vi "Trajectory Box Monitor.vi"() -> ()   [LabVIEW 2017]
uses:
  TCP/TCP Host/Controls/Host- Queue States.ctl
  TCP/TCP Host/Controls/Control - Testscreen.ctl
  Controls/Testscreen_Input cluster.ctl
  <vilib>/addons/database/Connection.llb/Conn ObjectReference.ctl
  Controls/Network_states.ctl
  TCP/TCP Engine/Controls/TCP - Driver Control.ctl
  Variable/Global 1.vi
  <vilib>/addons/database/Connection.llb/DB Tools Open Connec (String).vi
  <vilib>/addons/database/NI_Database_API.lvlib
panel:
  out "error out":errorcluster
  out "array":string[](array[string])
  out "Test Running":bool
  in  "DataLog Duration":string="00:01:27"
  in  "Exit":bool
  in  "Report":bool
  in  "Settings":bool
  in  "Test Screen":bool
  in  "ID Status":string
  in  "?":enum32{"Option A", "Option B"}(tab)
  in  "Test Profile":T1(array[cluster])=[{"Ram Up Time"=10.0, "Hold Time"=5.0, "Ramp Down"=10.0, "Concentration Value"=25.0}, {"Ram Up Time"=15.0, "Hold Time"=10.0, "Ramp Down"=5.0, "Concentration Value"=35.0}, {"Ram Up Time"=0.0, "Hold Time"=0.0, "Ramp Down"=0.0, "Concentration Value"=0.0}]
  out "Profile Plotting":cluster{"X":dbl, "Y":dbl}[](graph)
  in  "Profile File Selection":u16(ring) items=["Test A", "Test B", "Test C"]
  in  "Iterations":dbl
  in  "Gas Selection":u16(ring) items=["Test A", "Test B", "Test C"]
  in  "Drive  2":string
  in  "Drive":string
  in  "IP Address":string
  in  "error in (no error)":errorcluster
  in  "Note":string
  in  "Tab- Main":enum32{"Settings", "Report", "Testscreen"}(tab)
  in  "Tab Control Testscreen 4":enum32{"Channel Mapping", "Test Settings"}(tab)
  in  "Channel Mapping":T2(array[cluster])
  in  "Sampling Frequency (Hz)":string="Trajectory"
  in  "Wifi Name":string="Trajectory"
  in  "Test Inactivity Time":dbl=30.0 format="%<%H:%M:%S>t"
  in  "Drive Path":path=path "D:/Trajectory Data"
  in  "cRIO IP Address":string="192.168.1.1"
  out "Test Time":dbl=1.0 format="%<%H:%M:%S>t"
  in  "Save Test Settings":bool
  in  "Tab Control Testscreen 5":enum32{"Report", "Detailed Report"}(tab)
  in  "Fetch Report":bool
  in  "To Date & Time":timestamp format="%<%x>T"
  in  "From Date & Time":timestamp format="%<%x>T"
  out "Report Data":i32(listbox)
  in  "Test Stop Time :":string="12:59:05"
  in  "Tab Control Testscreen 6":enum32{"Data", "Histogram"}(tab)
  in  "Report Data 2":i32(listbox)
  out "XY Graph 3":cluster{i32, "Numeric":u16}[](graph)
  in  "ID Status :":string="00068OK"
  in  "ID :":string="Trajectory"
  in  "Angle :":string="Multi"
  in  "Flow :":string="Flow"
  in  "Material :":string="Cole"
  in  "Furnace :":string="G Furnace"
  in  "Test Start Time:":string="12:59:05"
  in  "Date :":string="02/07/2021"
  out "Date":string
  in  "Tab- Main 2":T3(tab)
  in  "Test details":T4={"Furnace"="Furnace A", "Material"="Coke", "Angle"="Multi Angle", "ID"="Trajectory 9", "Flowrate"="Flow", "Test Name"="Coke Burn", "Tested By"="Anirban"}
  in  "Save Test Info":bool
  out "Data Logging Path":path
  in  "Probe 2":bool[](array[boolean])=[TRUE, FALSE, FALSE, FALSE, TRUE, FALSE, FALSE, FALSE, FALSE, FALSE, FALSE, FALSE, FALSE, FALSE, FALSE, FALSE, FALSE, FALSE, FALSE, FALSE, FALSE, FALSE, FALSE, FALSE, FALSE, FALSE, FALSE, FALSE, FALSE, FALSE, FALSE, FALSE, FALSE, FALSE, FALSE, FALSE, FALSE, FALSE, FALSE, FALSE, FALSE, FALSE, FALSE, FALSE, FALSE, FALSE, FALSE, FALSE, FALSE, FALSE, FALSE, FALSE, FALSE, FALSE, FALSE, FALSE, FALSE, FALSE, FALSE, FALSE]
  in  "Probe":bool[](array[boolean])
  in  "Probe 3":bool[](array[boolean])=[TRUE, FALSE, FALSE, FALSE, TRUE, FALSE, FALSE, FALSE, FALSE, FALSE, FALSE, FALSE, FALSE, FALSE, FALSE, FALSE, FALSE, FALSE, FALSE, FALSE, FALSE, FALSE, FALSE, FALSE, FALSE, FALSE, FALSE, FALSE, FALSE, FALSE, FALSE, FALSE, FALSE, FALSE, FALSE, FALSE, FALSE, FALSE, FALSE, FALSE, FALSE, FALSE, FALSE, FALSE, FALSE, FALSE, FALSE, FALSE, FALSE, FALSE, FALSE, FALSE, FALSE, FALSE, FALSE, FALSE, FALSE, FALSE, FALSE, FALSE]
  out "XY Graph":cluster{i32, "Numeric":i32}[](graph)
  in  "Setup":bool
  out "Datalog Duration":dbl format="%<%H:%M:%S>t"
  in  "Disk Space Host":string="Trajectory 9"
  in  "Disk Space cRIO":string="Trajectory 9"
  in  "Calibrations":bool
  in  "Alarms":i32(listbox)
  out "Wifi":bool=TRUE
  out "Logging 3":bool=TRUE
  in  "Start Test":bool
  in  "Stop Test":bool
  out "Message":string="Acquiring Data"
  # "Test Setup Setting"
  # "Trajectory Box Monitor System"
  # "Trajectory Box Monitor"
  # "1"
  # "5"
  # "10"
  # "15"
  # "20"
  # "41"
  # "45"
  # "50"
  # "55"
  # "60"
  # "21"
  # "25"
  # "30"
  # "40"
  # "35"
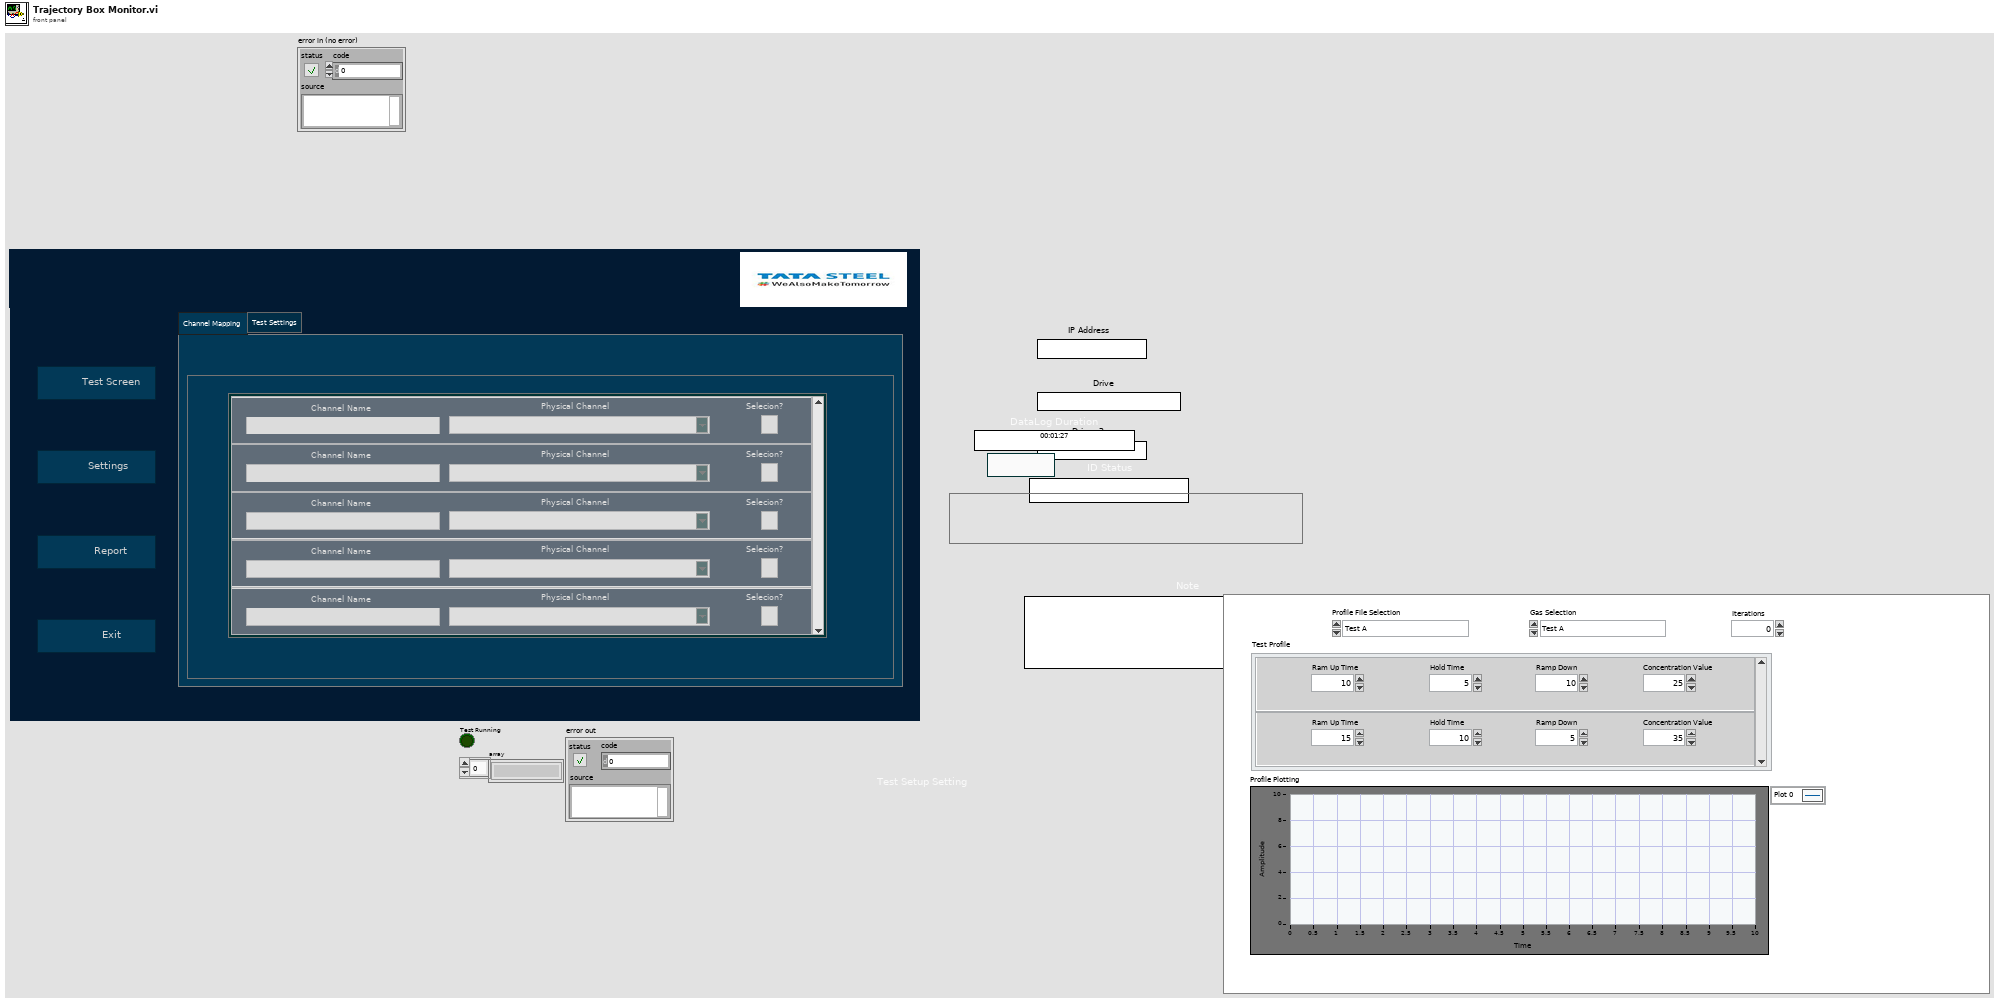
[diagram p1: front panel]
types:
  T1 = cluster{"Ram Up Time":dbl, "Hold Time":dbl, "Ramp Down":dbl, "Concentration Value":dbl}[]
  T2 = cluster{"Channel Name":string, " Physical Channel":tag, "Selecion?":bool}[]
  T3 = enum32{"Test Information", "Sensor Status", "Histogram", "Info", "Software Log"}
  T4 = cluster{"Furnace":string, "Material":string, "Angle":string, "ID":string, "Flowrate":string, "Test Name":string, "Tested By":string}
  T5 = typedef "Network_states.ctl" = enum16{"Connect", "Transfer Files", "Close"}
  T6 = typedef "Testscreen_Input cluster.ctl" = cluster{"Message":string, "Histogram Data":i32[], "Timer 1":u32, "Test Running":bool, "connection reference":T7}
  T7 = typedef "NI_Database_API.lvlib/Conn ObjectReference.ctl" = refnum<k1>
  T8 = typedef "Control - Testscreen.ctl" = enum16{"No Event", "Init", "Download Files", "Test Running", "Update Test Results", "Machine Unhealthy", "Autotest Started", "Test Aborted", "Sequence Complete", "Update Sensor Data", "Log File Available", "Machine Mode", "Aux Logging Started", "Aux File Saved", "Get PID Values", "View Report", "Exit", "Wait", "Abort", "Copy Log File", "Generate Alarm", "Send Test Details"}
  T9 = typedef "Host- Queue States.ctl" = enum16{"Initialize", "Enqueue", "Enqueue Priority", "Dequeue", "Flush", "Destroy"}
  T10 = cluster{"Test details":cluster{"Furnace":string, "Material":string, "Angle":string, "ID":string, "Flowrate":string, "Test Name":string, "Tested By":string}, "Datalog Duration":dbl}
  T11 = typedef "TCP - Driver Control.ctl" = enum16{"Test Settings", "Boolean Commands", "Test Results", "Send Test Details"}
  T12 = cluster{"Channel Name":string, " Physical Channel":tag, "Selecion?":bool}
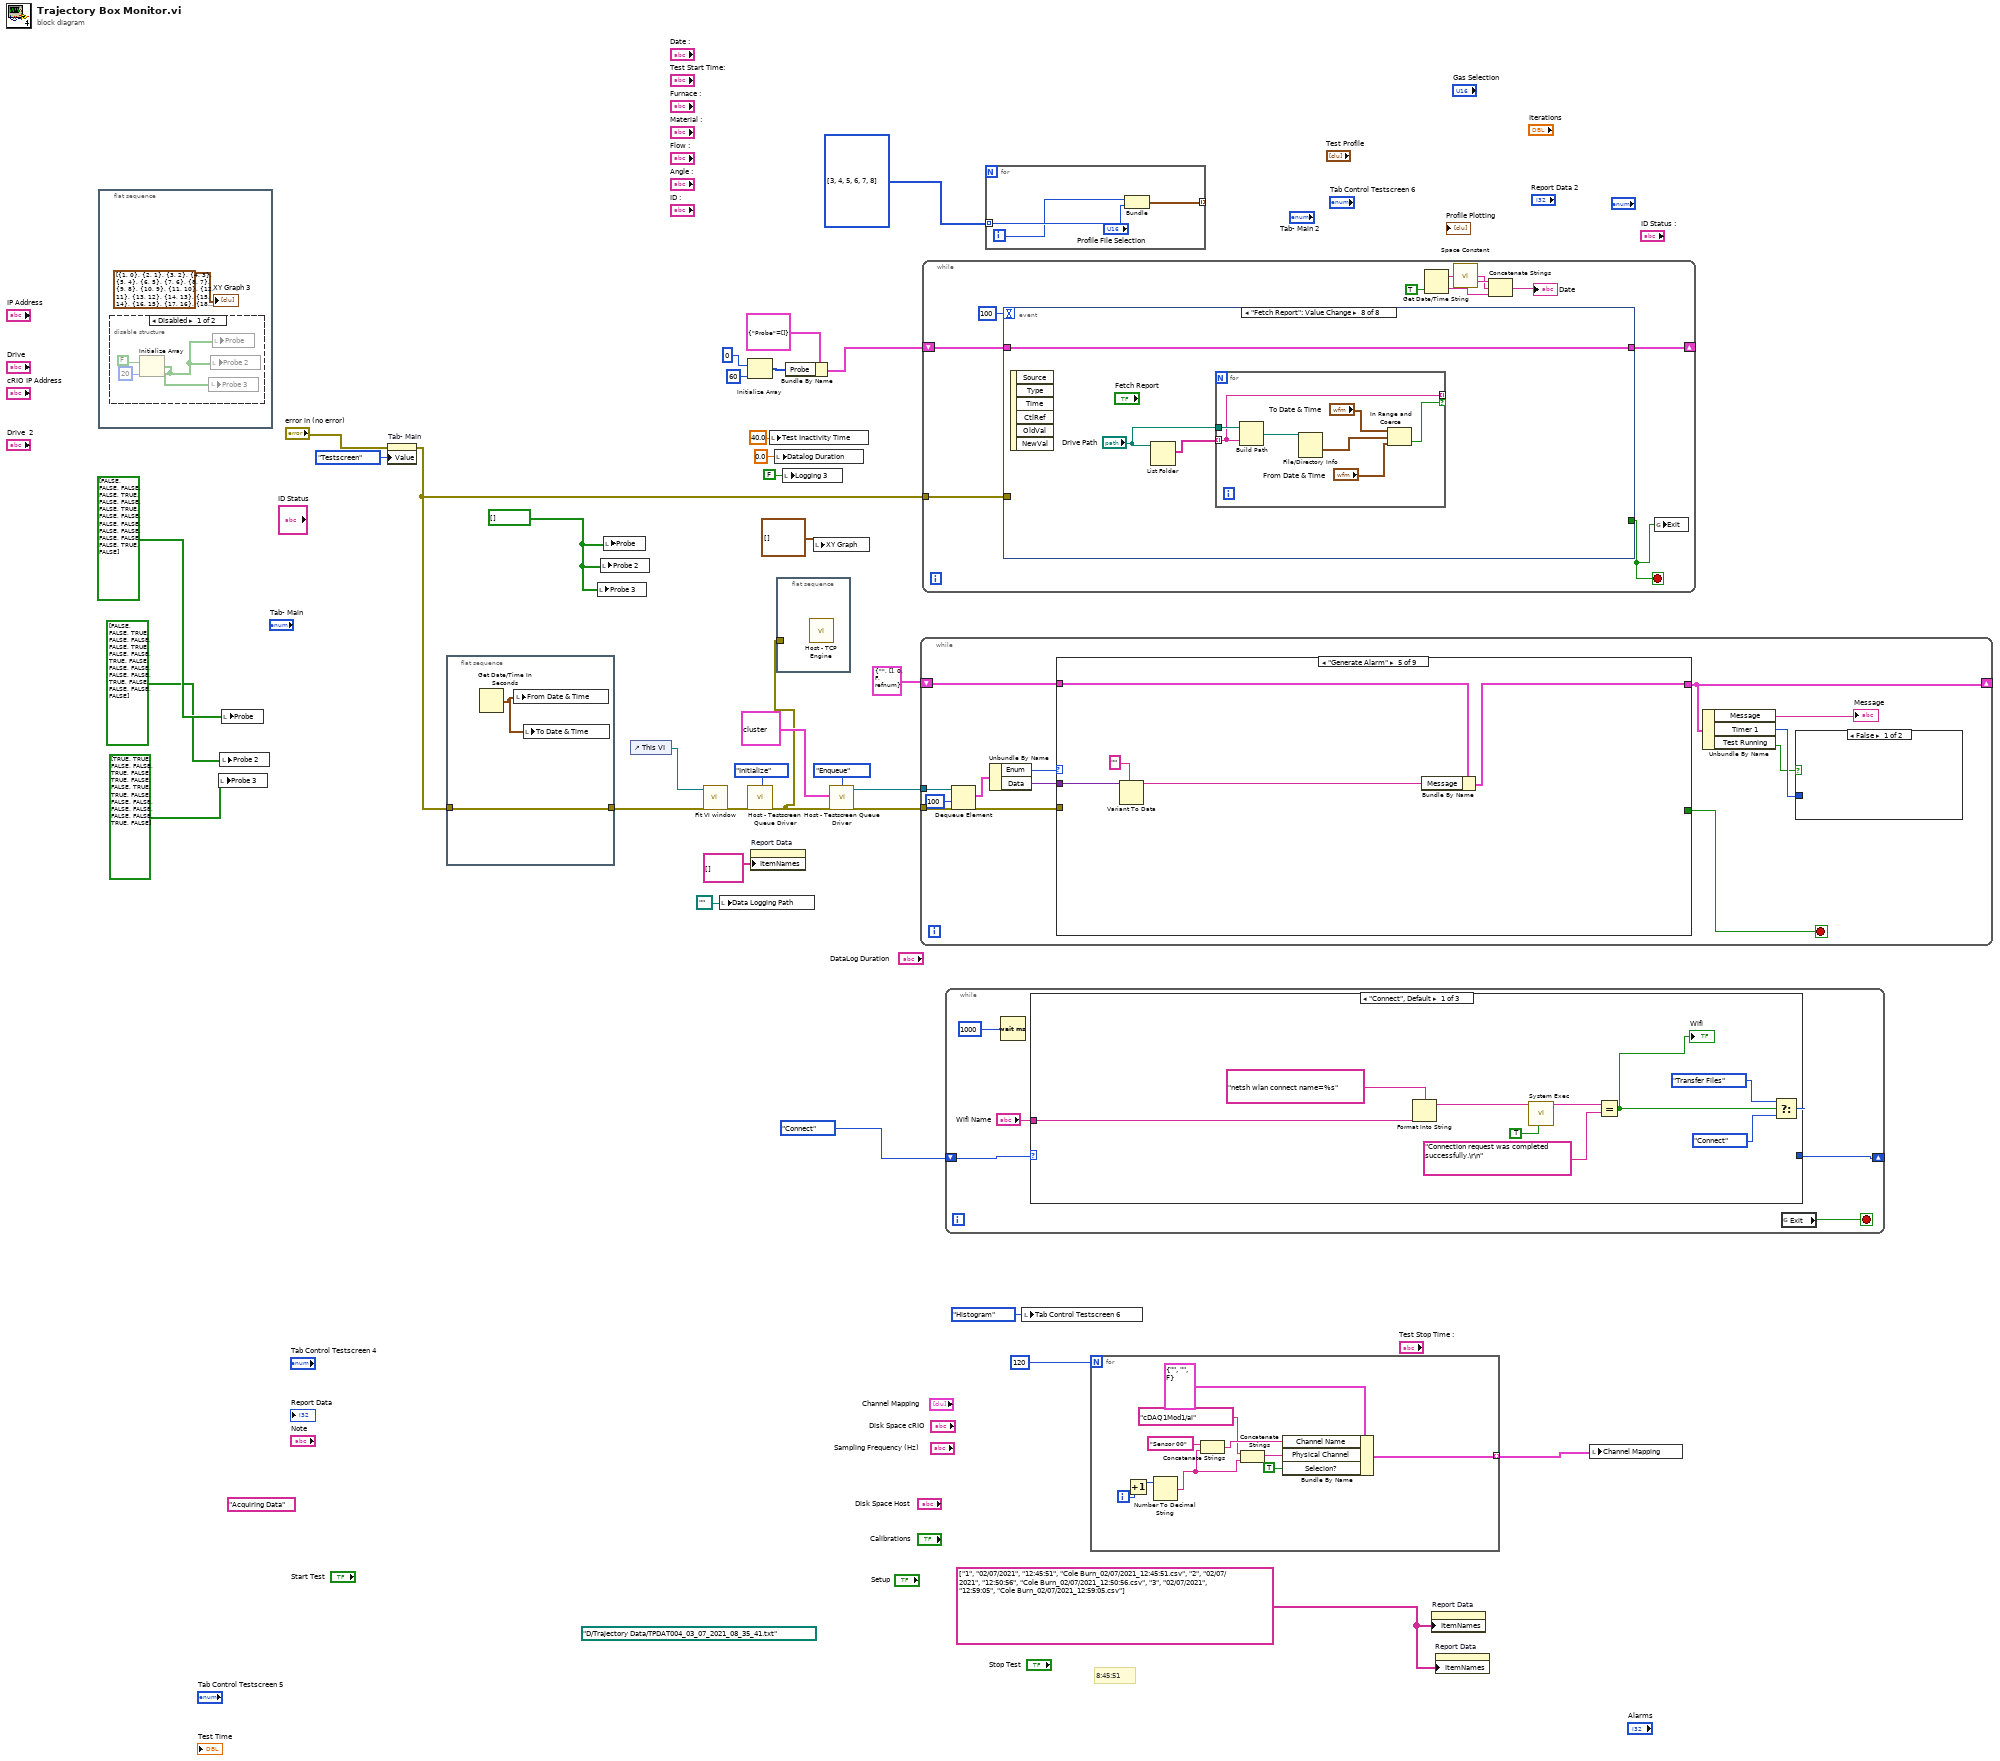
[diagram p0: block diagram]
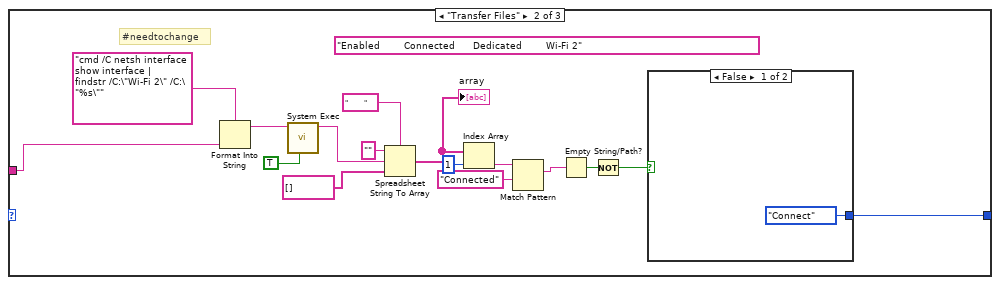
[diagram p2: hidden frame]
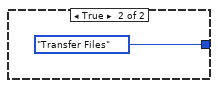
[diagram p3: hidden frame]
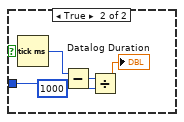
[diagram p5: hidden frame]
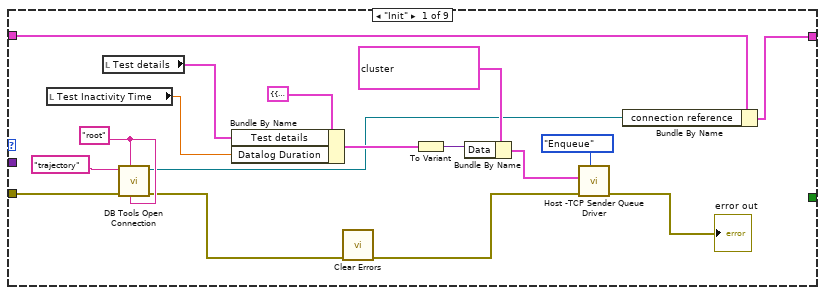
[diagram p6: hidden frame]
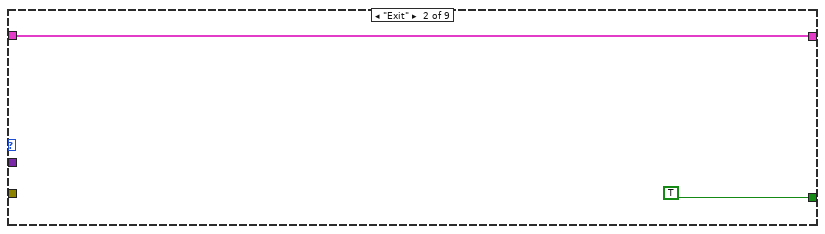
[diagram p7: hidden frame]
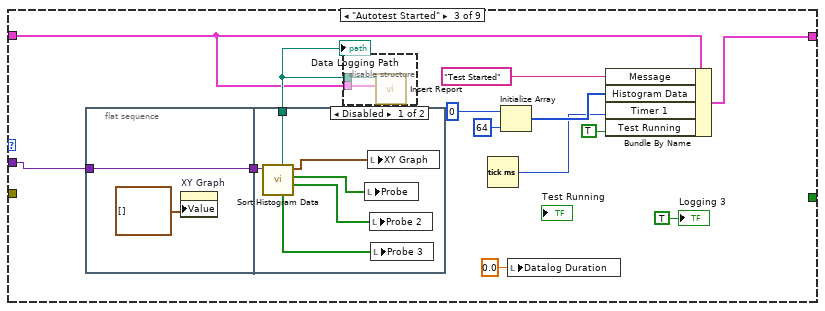
[diagram p8: hidden frame]
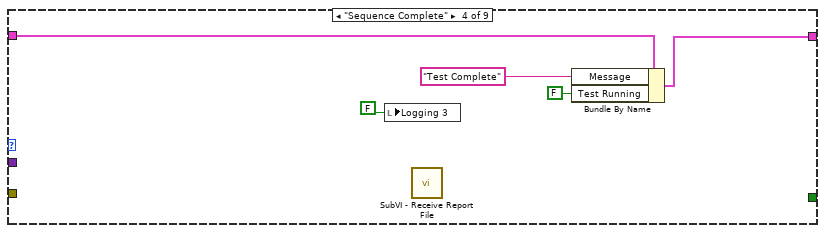
[diagram p10: hidden frame]
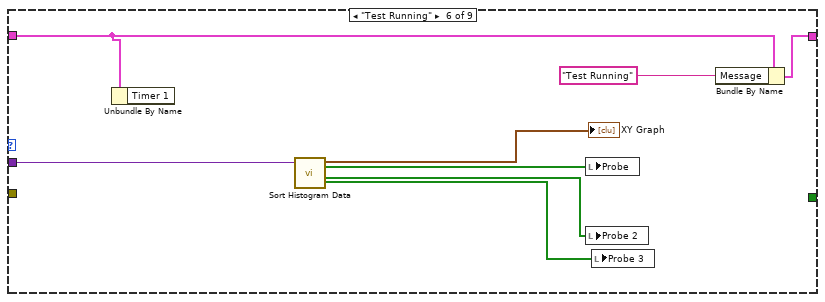
[diagram p11: hidden frame]
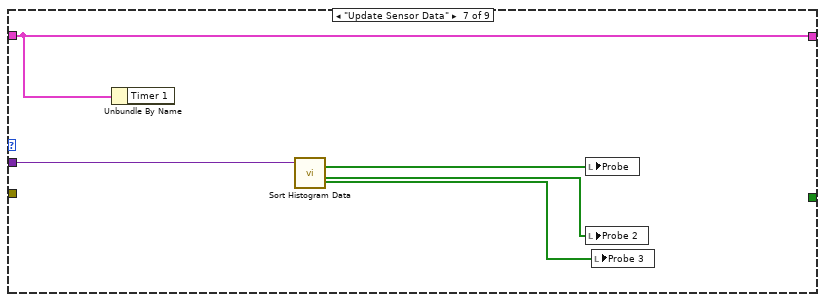
[diagram p12: hidden frame]
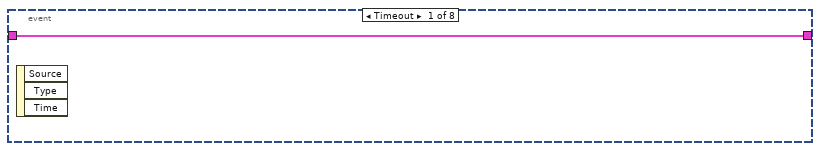
[diagram p16: hidden frame]
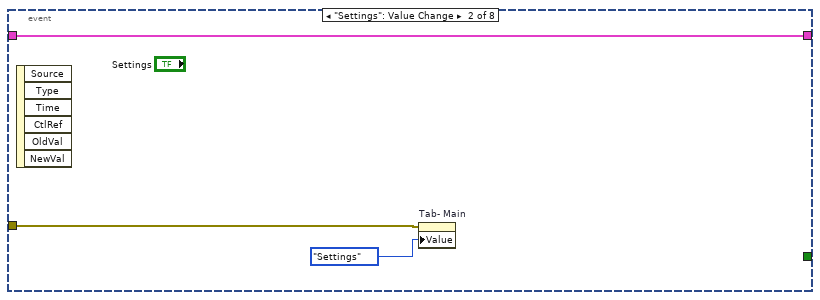
[diagram p17: hidden frame]
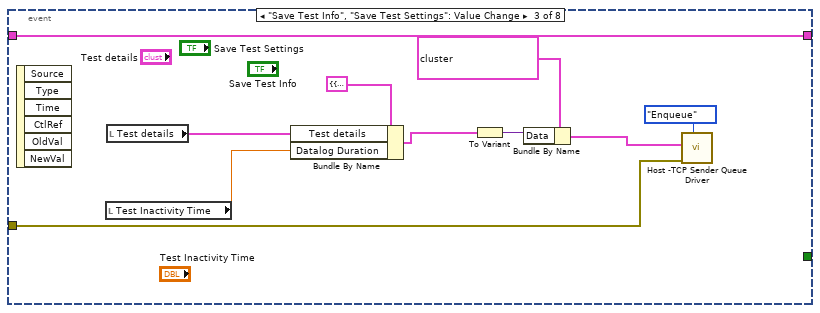
[diagram p18: hidden frame]
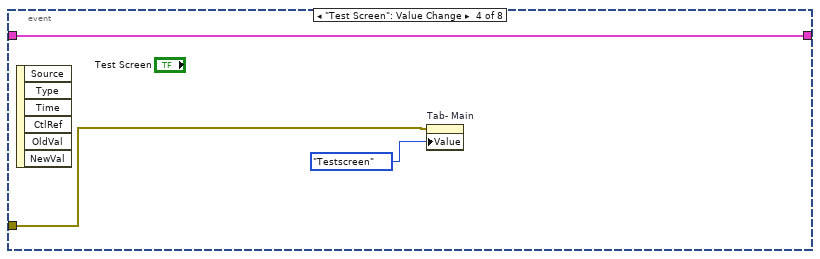
[diagram p19: hidden frame]
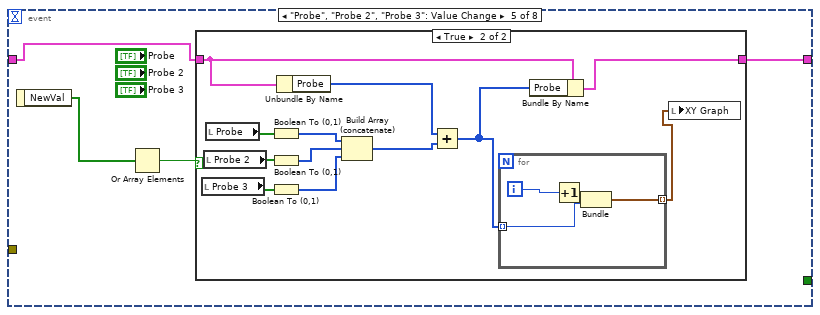
[diagram p20: hidden frame]
diagram:
  w13 = bool[] [] ("Probe")
  w20 = string[][] [["1", "02/07/2021", "12:45:51", "Cole Burn_02/07/2021_12:45:51.csv"], ["2", "02/07/2021", "12:50:56", "Cole Burn_02/07/2021_12:50:56.csv"], ["3", "02/07/2021", "12:59:05", "Cole Burn_02/07/2021_12:59:05.csv"]] ("Item Names")
  (unwired) path "D:/Trajectory Data/TPDAT004_03_07_2021_08_35_41.txt" ("Data Logging Path")
  (unwired) "Acquiring Data" ("Message")
  # "8:45:51"
  n1 = flat-sequence {
    frame #0 {
      n2 = disable-structure shown="Disabled" {
        frame Disabled {
          n3 = Initialize Array(FALSE ("Boolean"), 20 ("dimension size")) -> (w36:bool[])
          n4 = local write "Probe 3"(w36) -> ()
          n5 = local write "Probe 2"(w36) -> ()
          n6 = local write "Probe"(w36) -> ()
        }
        frame Enabled {
        }
      }
      "XY Graph 3" <- cluster{i32, "Numeric":u16}[] [{1, "Numeric"=0}, {2, "Numeric"=1}, {3, "Numeric"=2}, {4, "Numeric"=3}, {5, "Numeric"=4}, {6, "Numeric"=5}, {7, "Numeric"=6}, {8, "Numeric"=7}, {9, "Numeric"=8}, {10, "Numeric"=9}, {11, "Numeric"=10}, {12, "Numeric"=11}, {13, "Numeric"=12}, {14, "Numeric"=13}, {15, "Numeric"=14}, {16, "Numeric"=15}, {17, "Numeric"=16}, {18, "Numeric"=17}, {19, "Numeric"=18}, {20, "Numeric"=19}, {21, "Numeric"=20}, {22, "Numeric"=21}, {23, "Numeric"=22}, {24, "Numeric"=23}, {25, "Numeric"=24}, {26, "Numeric"=25}, {27, "Numeric"=26}, {28, "Numeric"=27}, {29, "Numeric"=28}, {30, "Numeric"=29}, {30, "Numeric"=29}, {31, "Numeric"=28}, {32, "Numeric"=27}, {33, "Numeric"=26}, {34, "Numeric"=25}, {35, "Numeric"=24}, {36, "Numeric"=23}, {37, "Numeric"=22}, {38, "Numeric"=21}, {39, "Numeric"=20}, {40, "Numeric"=19}, {41, "Numeric"=18}, {42, "Numeric"=17}, {43, "Numeric"=16}, {44, "Numeric"=15}, {45, "Numeric"=14}, {46, "Numeric"=13}, {47, "Numeric"=12}, {48, "Numeric"=11}, {49, "Numeric"=10}, {50, "Numeric"=9}, {51, "Numeric"=8}, {52, "Numeric"=7}, {53, "Numeric"=6}, {54, "Numeric"=5}, {55, "Numeric"=4}, {56, "Numeric"=3}, {57, "Numeric"=2}, {58, "Numeric"=1}, {59, "Numeric"=0}] ("appended array 2")
    }
  }
  n7 = local write "Probe 3"(bool[] [TRUE, TRUE, FALSE, FALSE, TRUE, FALSE, TRUE, FALSE, FALSE, TRUE, TRUE, FALSE, FALSE, FALSE, FALSE, FALSE, FALSE, FALSE, TRUE, FALSE] ("Probe")) -> ()
  n8 = local write "Probe 2"(bool[] [FALSE, FALSE, TRUE, FALSE, FALSE, FALSE, TRUE, FALSE, FALSE, TRUE, FALSE, FALSE, FALSE, FALSE, FALSE, TRUE, FALSE, FALSE, FALSE, FALSE] ("Probe")) -> ()
  n9 = local write "Probe"(bool[] [FALSE, FALSE, FALSE, FALSE, TRUE, FALSE, FALSE, FALSE, TRUE, FALSE, FALSE, FALSE, FALSE, FALSE, FALSE, FALSE, FALSE, FALSE, TRUE, FALSE] ("Probe")) -> ()
  n10 = property on="Tab- Main" class="TabCtl (strict)"(error in="error in (no error)", "Value"=enum32{"Settings", "Report", "Testscreen"}."Testscreen" ("Tab- Main")) -> (error out=w4:errorcluster)  [unwired: 1 in, 1 out]
  n11 = flat-sequence {
    tunnel: [w40] -> w3
    tunnel: w4 -> [w40]
    frame #0 {
      n12 = Get Date/Time In Seconds() -> (seconds since 1Jan1904=w39:timestamp)
      n13 = local write "From Date & Time"(w39) -> ()
      n14 = local write "To Date & Time"(w39) -> ()
    }
  }
  n15 = local write "Probe 3"(w13) -> ()
  n16 = local write "Probe 2"(w13) -> ()
  n17 = local write "Probe"(w13) -> ()
  n18 = control-ref of="This VI"() -> (w9:refnum<vi>)
  n19 = call "Fit VI window.vi"("error in (no error)"=w3, "VI Ref (calling VI)"=w9) -> ("error out"=w10:errorcluster)  [unwired: 9 in]
  n20 = local write "Data Logging Path"(path "" ("Data Logging Path")) -> ()
  n21 = Initialize Array(0 ("Numeric"), 60 ("dimension size")) -> (w30:i32[])
  n22 = call "Host - Testscreen Queue Driver.vi"("Cases"=Host-_Queue_States."Initialize", "error in (no error)"=w10) -> ("error out"=w1:errorcluster)  [unwired: 7 in, 2 out]
  n23 = property on="Report Data" class="MCListbox (strict)"("ItemNames"=string[][] [] ("Item Names")) -> ()  [unwired: 2 in, 2 out]
  n24 = local write "Test Inactivity Time"(40.0 ("Datalog Duration")) -> ()
  n25 = local write "Datalog Duration"(0.0 ("Datalog Duration")) -> ()
  n26 = flat-sequence {
    tunnel: w1 -> [_]
    frame #0 {
      n27 = call "Host - TCP Engine.vi"() -> ()  [unwired: 12 in]
    }
  }
  n28 = local write "Logging 3"(FALSE ("Logging 3")) -> ()
  n29 = Bundle By Name(cluster=cluster{"Probe":i32[]} {"Probe"=[]}, "Probe"=w30) -> (w28:cluster{"Probe":i32[]})
  n30 = local write "XY Graph"(cluster{i32, "Numeric":i32}[] [] ("XY Graph")) -> ()
  n31 = call "Host - Testscreen Queue Driver.vi"("Cases"=Host-_Queue_States."Enqueue", "error in (no error)"=w1, "Element In"=cluster{"Data":variant, "Enum":T8} {"Data"=variant, "Enum"=enum."Init"}) -> ("error out"=w15:errorcluster, "queue out"=w17:refnum<queue>)  [unwired: 6 in, 1 out]
  n32 = while {
    tunnel: w15 -> [w51]
    tunnel: w17 -> [w52]
    shift-right: [w46] -> _
    shift-left: T6 {"Message"="", "Histogram Data"=[], "Timer 1"=0, "Test Running"=FALSE, "connection reference"=refnum} -> [w47]
    stop <- w53 stop-if-true
    n33 = Dequeue Element(queue=w52, timeout in ms (-1)=100, error in (no error)=w51) -> (element=w49:cluster{"Data":variant, "Enum":T8}, error out=w50:errorcluster)  [unwired: 2 out]
    n34 = Unbundle By Name(w49) -> ("Enum"=w48:T8, "Data"=w44:variant)
    n35 = case shown="\"Generate Alarm\"" w48 {
      tunnel: w50 -> [w65 _ _ _ _ _ _ _ _]
      tunnel: [_ TRUE _ _ _ _ _ _ _] -> w53
      tunnel: w47 -> [w62 w76 w78 w105 w107 w111 w119 w124 w125]
      tunnel: [w61 w76 w89 w103 w106 w114 w119 w124 w125] -> w46
      tunnel: w44 -> [_ _ w85 _ w110 w118 w123 _ _]
      frame "Init" {
        w66 = "root" ("userID")
        n36 = local read "Test Inactivity Time"() -> (w68:dbl)
        n37 = local read "Test details"() -> (w70:T4)
        n38 = call-poly <vilib>:"DB Tools Open Connection.vi"("password"=w66, "userID"=w66, "error in (no error)"=w65, "connection information"="trajectory") -> ("error out"=w64:errorcluster, "connection reference"=w63:T7)  [unwired: 4 in]
        n39 = Bundle By Name(cluster=T10 {"Test details"={"Furnace"="Furnace A", "Material"="Aluminium", "Angle"="Multi Angle", "ID"="Trajectory 9", "Flowrate"="Flow", "Test Name"="Coke Burn", "Tested By"="Anirban"}, "Datalog Duration"=0.0}, "Test details"=w70, "Datalog Duration"=w68) -> (w69:T10)
        n40 = call <vilib>:"Clear Errors.vi"("error in (no error)"=w64) -> ("error out"=w60:errorcluster)  [unwired: 5 in, 1 out]
        n41 = To Variant(anything=w69) -> (Variant=w72:variant)
        n42 = Bundle By Name(cluster=cluster{"Data":variant, "State":T11} {"Data"=variant, "State"=enum."Send Test Details"} ("Element In"), "Data"=w72) -> (w75:cluster{"Data":variant, "State":T11})
        n43 = call "Host -TCP Sender Queue Driver.vi"("Cases"=Host-_Queue_States."Enqueue", "error in (no error)"=w60, "Element In"=w75) -> ("error out"=→"error out":errorcluster)  [unwired: 6 in, 2 out]
        n44 = Bundle By Name(cluster=w62, "connection reference"=w63) -> (w61:T6)
      }
      frame "Exit" {
      }
      frame "Autotest Started" {
        n45 = flat-sequence {
          tunnel: w85 -> [w94]
          tunnel: [w94] -> w84
          tunnel: w84 -> [w100]
          tunnel: [w95] -> w79
          frame #0 {
            n46 = property on="XY Graph" class="XYGraph (strict)"("Value"=cluster{i32, "Numeric":u16}[] [] ("XY Graph")) -> ()  [unwired: 2 in, 2 out]
          }
          frame #1 {
            n47 = call "Sort Histogram Data.vi"("Data"=w100) -> ("Array 2"=w97:bool[], "Array 3"=w98:bool[], "XY Graph"=w99:cluster{i32, "Numeric":i32}[], "Array"=w96:bool[], "File Path"=w95:path)  [unwired: 6 in]
            n48 = local write "Probe"(w98) -> ()
            n49 = local write "XY Graph"(w99) -> ()
            n50 = local write "Probe 2"(w97) -> ()
            n51 = local write "Probe 3"(w96) -> ()
          }
        }
        n52 = disable-structure shown="Disabled" {
          disable-tunnel: w79 -> [w92 _]
          disable-tunnel: w78 -> [w91 _]
          frame Disabled {
            n53 = call "Insert Report.vi"("Cluster"=w91, "Path"=w92) -> ()  [unwired: 9 in, 1 out]
          }
          frame Enabled {
          }
        }
        n54 = Tick Count (ms)() -> (millisecond timer value=w83:u32)
        n55 = Initialize Array(0, 64 ("dimension size")) -> (w86:i32[])
        n56 = local write "Datalog Duration"(0.0 ("Datalog Duration")) -> ()
        n57 = Bundle By Name(cluster=w78, "Message"="Test Started", "Histogram Data"=w86, "Timer 1"=w83, "Test Running"=TRUE) -> (w89:T6)
        "Data Logging Path" <- w79
        "Logging 3" <- TRUE ("Logging 3")
      }
      frame "Sequence Complete" {
        n58 = local write "Logging 3"(FALSE ("Logging 3")) -> ()
        n59 = call "SubVI - Receive Report File.vi"() -> ()  [unwired: 11 in, 1 out]
        n60 = Bundle By Name(cluster=w105, "Message"="Test Complete", "Test Running"=FALSE) -> (w103:T6)
      }
      frame "Generate Alarm" {
        n61 = Variant To Data(type="", Variant=w110) -> (data=w108:string)  [unwired: 1 in, 1 out]
        n62 = Bundle By Name(cluster=w107, "Message"=w108) -> (w106:T6)
      }
      frame "Test Running" {
        n63 = Unbundle By Name(w111) -> ()  [unwired: 1 out]
        n64 = call "Sort Histogram Data.vi"("Data"=w118) -> ("Array 2"=w116:bool[], "Array 3"=w117:bool[], "XY Graph"=→"XY Graph":cluster{i32, "Numeric":i32}[], "Array"=w115:bool[])  [unwired: 6 in, 1 out]
        n65 = local write "Probe"(w117) -> ()
        n66 = local write "Probe 2"(w116) -> ()
        n67 = local write "Probe 3"(w115) -> ()
        n68 = Bundle By Name(cluster=w111, "Message"="Test Running") -> (w114:T6)
      }
      frame "Update Sensor Data" {
        n69 = Unbundle By Name(w119) -> ()  [unwired: 1 out]
        n70 = call "Sort Histogram Data.vi"("Data"=w123) -> ("Array 2"=w121:bool[], "Array 3"=w122:bool[], "Array"=w120:bool[])  [unwired: 6 in, 2 out]
        n71 = local write "Probe"(w122) -> ()
        n72 = local write "Probe 2"(w121) -> ()
        n73 = local write "Probe 3"(w120) -> ()
      }
      frame "No Event", Default {
      }
      frame "Update Test Results" {
      }
    }
    n74 = Unbundle By Name(w46) -> ("Message"=→"Message":string, "Timer 1"=w43:u32, "Test Running"=w42:bool)
    n75 = case shown="False" w42 {
      tunnel: w43 -> [_ w57]
      frame False {
      }
      frame True {
        n76 = Tick Count (ms)() -> (millisecond timer value=w58:u32)
        n77 = Subtract(x=w58, y=w57) -> (x-y=w56:u32)
        n78 = Divide(x=w56, y=u32 1000) -> (x/y=→"Datalog Duration":dbl)
      }
    }
  }
  n79 = while {
    tunnel: w4 -> [w135]
    shift-right: [w133] -> _
    shift-left: w28 -> [w134]
    stop <- w126 stop-if-true
    n80 = event shown="[7] \"Fetch Report\": Value Change" {
      selector: _ -> [_ _ _ _ _ _ _ _]
      dyn-events: _ -> [_ _ _ _ _ _ _ _]
      timeout: 100 -> [_ _ _ _ _ _ _ _]
      tunnel: [_ _ _ _ _ _ TRUE _] -> w126
      tunnel: w135 -> [_ w139 w140 w152 _ w176 w177 _]
      tunnel: w134 -> [w136 w138 w149 w151 w154 w175 w180 w184]
      tunnel: [w136 w138 w149 w151 w153 w175 w180 w184] -> w133
      event Timeout {
        n81 = event-data() -> ()  [unwired: 1 in, 3 out]
      }
      event "Settings": Value Change {
        n82 = event-data() -> ()  [unwired: 1 in, 6 out]
        n83 = property on="Tab- Main" class="TabCtl (strict)"(error in=w139, "Value"=enum32{"Settings", "Report", "Testscreen"}."Settings" ("Tab- Main")) -> ()  [unwired: 1 in, 2 out]
      }
      event "Save Test Info", "Save Test Settings": Value Change {
        n84 = event-data() -> ()  [unwired: 1 in, 6 out]
        n85 = local read "Test Inactivity Time"() -> (w148:dbl)
        n86 = local read "Test details"() -> (w146:T4)
        n87 = Bundle By Name(cluster=T10 {"Test details"={"Furnace"="Furnace A", "Material"="Aluminium", "Angle"="Multi Angle", "ID"="Trajectory 9", "Flowrate"="Flow", "Test Name"="Coke Burn", "Tested By"="Anirban"}, "Datalog Duration"=0.0}, "Test details"=w146, "Datalog Duration"=w148) -> (w147:T10)
        n88 = To Variant(anything=w147) -> (Variant=w144:variant)
        n89 = Bundle By Name(cluster=cluster{"Data":variant, "State":T11} {"Data"=variant, "State"=enum."Send Test Details"} ("Element In"), "Data"=w144) -> (w141:cluster{"Data":variant, "State":T11})
        n90 = call "Host -TCP Sender Queue Driver.vi"("Cases"=Host-_Queue_States."Enqueue", "error in (no error)"=w140, "Element In"=w141) -> ()  [unwired: 6 in, 3 out]
      }
      event "Test Screen": Value Change {
        n91 = event-data() -> ()  [unwired: 1 in, 6 out]
        n92 = property on="Tab- Main" class="TabCtl (strict)"(error in=w152, "Value"=enum32{"Settings", "Report", "Testscreen"}."Testscreen" ("Tab- Main")) -> ()  [unwired: 1 in, 2 out]
      }
      event "Probe", "Probe 2", "Probe 3": Value Change {
        n93 = event-data() -> ("NewVal"=w156:bool[])  [unwired: 1 in]
        n94 = Or Array Elements(Boolean array=w156) -> (logical OR=w155:bool)
        n95 = case shown="True" w155 {
          tunnel: w154 -> [w157 w160]
          tunnel: [w157 w159] -> w153
          frame False {
          }
          frame True {
            n96 = local read "Probe 3"() -> (w167:bool[])
            n97 = local read "Probe 2"() -> (w168:bool[])
            n98 = local read "Probe"() -> (w169:bool[])
            n99 = Boolean To (0,1)(Boolean=w169) -> (0, 1=w166:i16[])
            n100 = Boolean To (0,1)(Boolean=w168) -> (0, 1=w165:i16[])
            n101 = Boolean To (0,1)(Boolean=w167) -> (0, 1=w164:i16[])
            n102 = Unbundle By Name(w160) -> ("Probe"=w163:i32[])
            n103 = Build Array (concatenate)(w166, w165, w164) -> (w162:i16[])
            n104 = Add(x=w163, y=w162) -> (x+y=w158:i32[])
            n105 = for {
              tunnel: [w173] -> w161 mode=indexing
              tunnel: w158 -> [w172] mode=indexing
              i -> [w171]
              n106 = Increment(x=w171) -> (x+1=w170:i32)
              n107 = Bundle(w170, w172) -> (w173:cluster{i32, i32})  [unwired: 1 in]
            }
            n108 = Bundle By Name(cluster=w160, "Probe"=w158) -> (w159:cluster{"Probe":i32[]})
            n109 = local write "XY Graph"(w161) -> ()
          }
        }
      }
      event "Report": Value Change {
        n110 = event-data() -> ()  [unwired: 1 in, 6 out]
        n111 = property on="Tab- Main" class="TabCtl (strict)"(error in=w176, "Value"=enum32{"Settings", "Report", "Testscreen"}."Report" ("Tab- Main")) -> ()  [unwired: 1 in, 2 out]
      }
      event "Exit": Value Change {
        n112 = event-data() -> ()  [unwired: 1 in, 6 out]
        n113 = call "Host - Testscreen Queue Driver.vi"("Cases"=Host-_Queue_States."Enqueue", "error in (no error)"=w177, "Element In"=cluster{"Data":variant, "Enum":T8} {"Data"=variant, "Enum"=enum."Exit"}) -> ()  [unwired: 6 in, 3 out]
      }
      event "Fetch Report": Value Change {
        n114 = event-data() -> ()  [unwired: 1 in, 6 out]
        n115 = List Folder(path="Drive Path") -> (filenames=w182:string[])  [unwired: 3 in, 3 out]
        n116 = for {
          tunnel: "Drive Path" -> [w191]
          tunnel: w182 -> [w186] mode=indexing
          tunnel: [w186] -> _ mode=indexing if=w185
          n117 = Build Path(base path=w191, name or relative path=w186) -> (appended path=w190:path)
          n118 = File/Directory Info(path=w190) -> (last mod=w189:timestamp)  [unwired: 1 in, 6 out]
          n119 = In Range and Coerce(upper limit="To Date & Time", x=w189, lower limit="From Date & Time") -> (In Range?=w185:bool)  [unwired: 1 out]
        }
      }
    }
    n120 = Get Date/Time String(want seconds? (F)=TRUE) -> (date string=w130:string, time string=w128:string)  [unwired: 2 in]
    n121 = call <vilib>:"Space Constant.vi"() -> ("String"=w129:string)
    n122 = Concatenate Strings(w130, w129, w128) -> (→"Date":string)
    n123 = global write "Global 1.vi" "Exit"(w126) -> ()
  }
  n124 = while {
    shift-right: [w194] -> _
    shift-left: Network_states."Connect" -> [w195]
    stop <- w196 stop-if-true
    n125 = Wait (ms)(milliseconds to wait=u32 1000) -> ()  [unwired: 1 out]
    n126 = case shown="\"Connect\", Default" w195 {
      tunnel: [w199 w207 _] -> w194
      tunnel: "Wifi Name" -> [w198 w219 _]
      frame "Connect", Default {
        n127 = Format Into String(format string="netsh wlan connect name=%s" ("command line"), w198) -> (resulting string=w202:string)  [unwired: 2 in, 1 out]
        n128 = call <vilib>:"System Exec.vi"("run minimized? (F)"=TRUE, "command line"=w202) -> ("standard output"=w205:string)  [unwired: 6 in, 3 out]
        n129 = Equal?(x=w205, y="Connection request was completed successfully.\r\n") -> (x = y?=w197:bool)
        "Wifi" <- w197
        n130 = Select(t=Network_states."Transfer Files", s=w197, f=Network_states."Connect") -> (s? t:f=w199:T5)
      }
      frame "Transfer Files" {
        (unwired) "Enabled        Connected      Dedicated        Wi-Fi 2" ("format string")
        # "#needtochange"
        n131 = Format Into String(format string="cmd /C netsh interface show interface | findstr /C:\"Wi-Fi 2\" /C:\"%s\"" ("command line"), w219) -> (resulting string=w221:string)  [unwired: 2 in, 1 out]
        n132 = call <vilib>:"System Exec.vi"("run minimized? (F)"=TRUE, "command line"=w221) -> ("standard output"=w217:string)  [unwired: 6 in, 3 out]
        n133 = Spreadsheet String To Array(delimiter (Tab)="        ", format string="", spreadsheet string=w217, array type (2D Dbl)=string[] []) -> (array=w214:string[])
        "array" <- w214
        n134 = Index Array(array=w214, index=1) -> (element=w212:string)
        n135 = Match Pattern(string=w212, regular expression="Connected") -> (match substring=w210:string)  [unwired: 1 in, 3 out]
        n136 = Empty String/Path?(string/path=w210) -> (empty?=w209:bool)
        n137 = Not(x=w209) -> (.not. x?=w208:bool)
        n138 = case shown="False" w208 {
          tunnel: [Network_states."Connect" Network_states."Transfer Files"] -> w207
          frame False {
          }
          frame True {
          }
        }
      }
      frame "Close" {
      }
    }
    n139 = global read "Global 1.vi" "Exit"() -> (w196:bool)
  }
  n140 = for {
    tunnel: [w227] -> _ mode=indexing
    tunnel: u16[] [3, 4, 5, 6, 7, 8] -> [w226] mode=indexing
    i -> [w225]
    n141 = Bundle(w225, "Numeric"=w226) -> (w227:cluster{i32, "Numeric":u16})  [unwired: 1 in]
  }
  n142 = local write "Tab Control Testscreen 6"(enum32{"Data", "Histogram"}."Histogram" ("Tab Control Testscreen 6")) -> ()
  n143 = for {
    N: 120 -> [_]
    tunnel: [w228] -> w22 mode=indexing
    i -> [w235]
    n144 = Increment(x=w235) -> (x+1=w231:i32)
    n145 = Number To Decimal String(number=w231) -> (decimal integer string=w232:string)  [unwired: 1 in]
    n146 = Concatenate Strings("Sensor 00" ("string"), w232) -> (w234:string)
    n147 = Concatenate Strings("cDAQ1Mod1/ai" ("string"), w232) -> (w230:string)
    n148 = Bundle By Name(cluster=T12 {"Channel Name"="", " Physical Channel"="", "Selecion?"=FALSE} ("Channel Mapping"), "Channel Name"=w234, "Physical Channel"=w230, "Selecion?"=TRUE) -> (w228:T12)
  }
  n149 = property on="Report Data" class="MCListbox (strict)"("ItemNames"=w20) -> ()  [unwired: 2 in, 2 out]
  n150 = property on="Report Data" class="MCListbox (strict)"("ItemNames"=w20) -> ()  [unwired: 2 in, 2 out]
  n151 = local write "Channel Mapping"(w22) -> ()
